vi "Config Sequence.vi"(8 "error in (no error)":errorcluster, 10 "new element/subarray":refnum<class "STEP.lvclass">, 11 "All Sequence STEPs in":refnum<class "STEP.lvclass">[](array[class])) -> (0 "error out":errorcluster, 3 "All Sequence STEPs":refnum<class "STEP.lvclass">[](array[class]))   [LabVIEW 2014, in "SeqLoop.lvlib"]
doc: "Configura las Mediciones."
uses:
  SeqLoop.lvlib
  Classes/STEP/STEP.lvclass
  <vilib>/regexp/Match Regular Expression.xnode
panel:
  in  "Ver Seq":bool
  in  "Stop Seq":bool
  in  "Delete Seq":bool
  in  "Add Seq":bool
  in  "Secuencias":i32(listbox)=-1 caption="Secuencia"
  in  "Edit Seq":bool
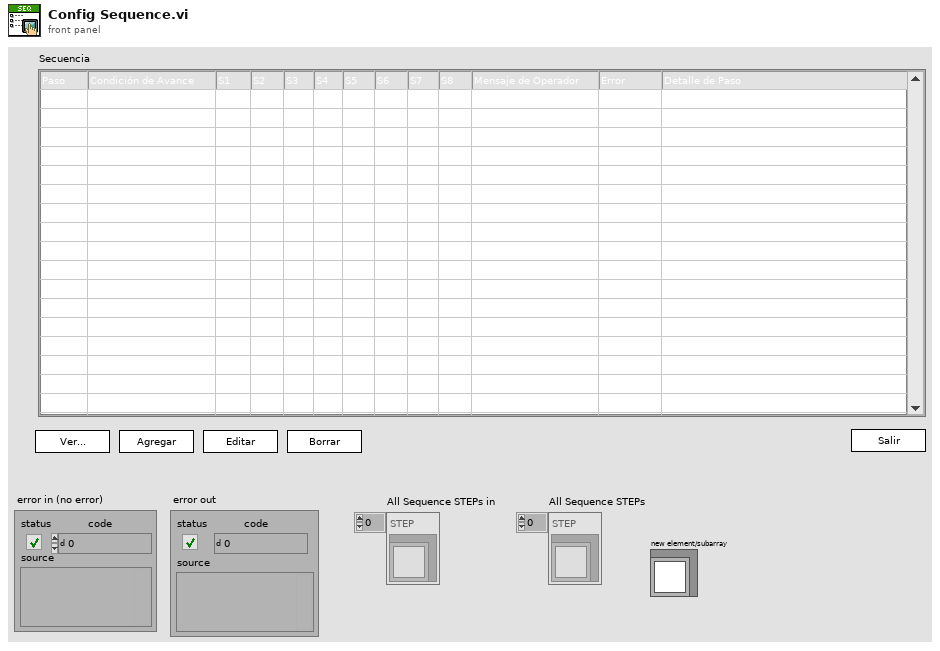
[diagram p1: front panel]
types:
  T1 = enum8{"Enabled", "Disabled", "Disabled and Grayed Out"}
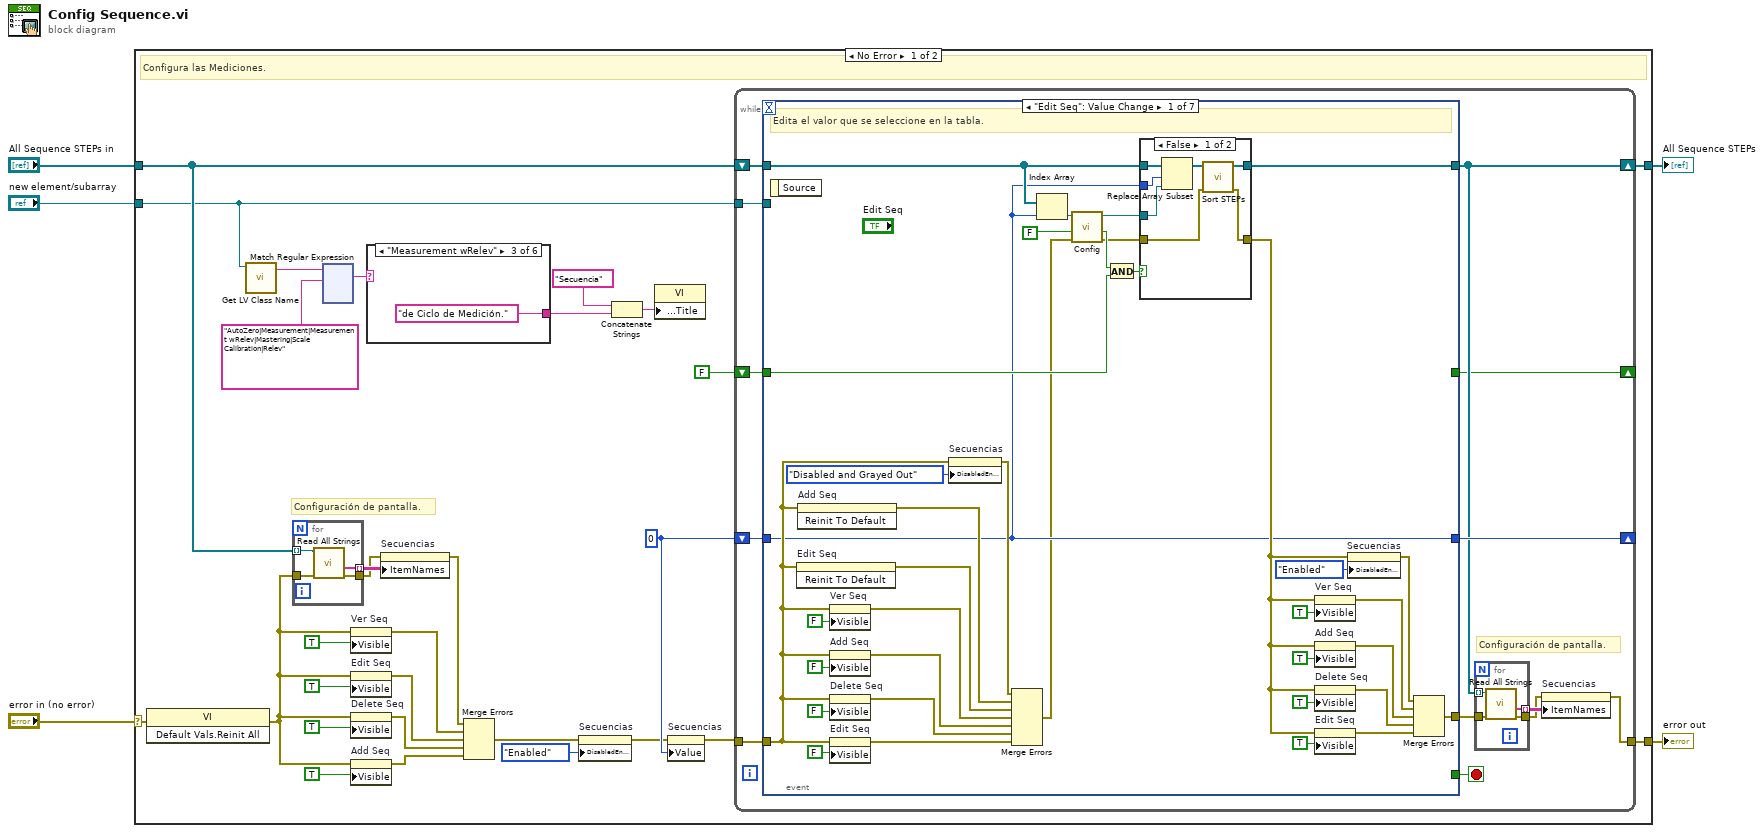
[diagram p0: block diagram]
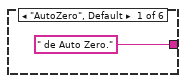
[diagram p2: hidden frame]
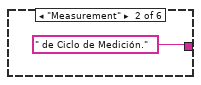
[diagram p3: hidden frame]
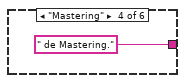
[diagram p4: hidden frame]
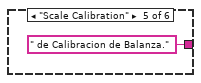
[diagram p5: hidden frame]
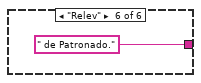
[diagram p6: hidden frame]
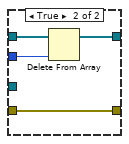
[diagram p7: hidden frame]
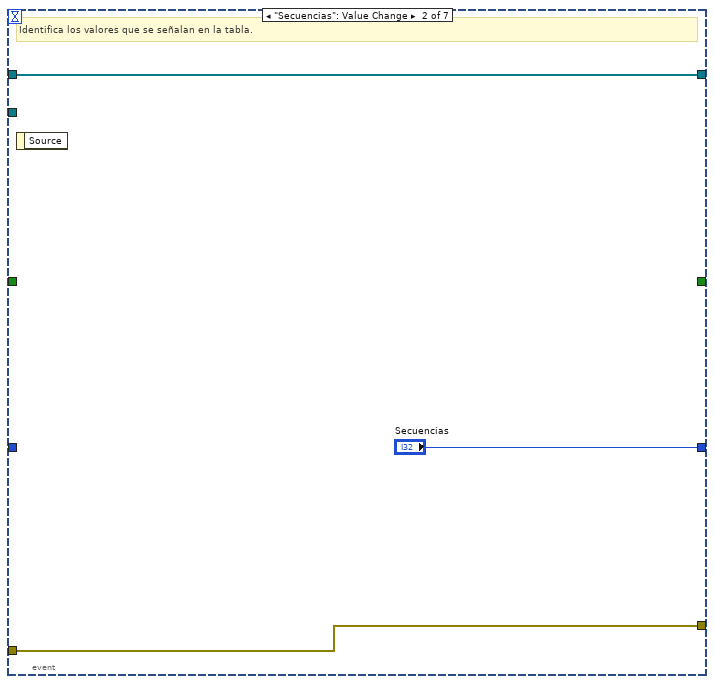
[diagram p8: hidden frame]
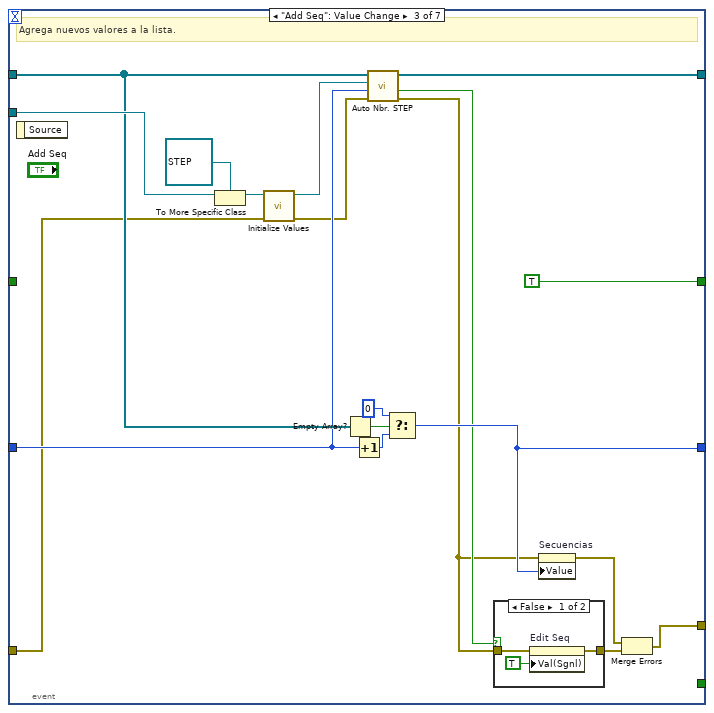
[diagram p9: hidden frame]
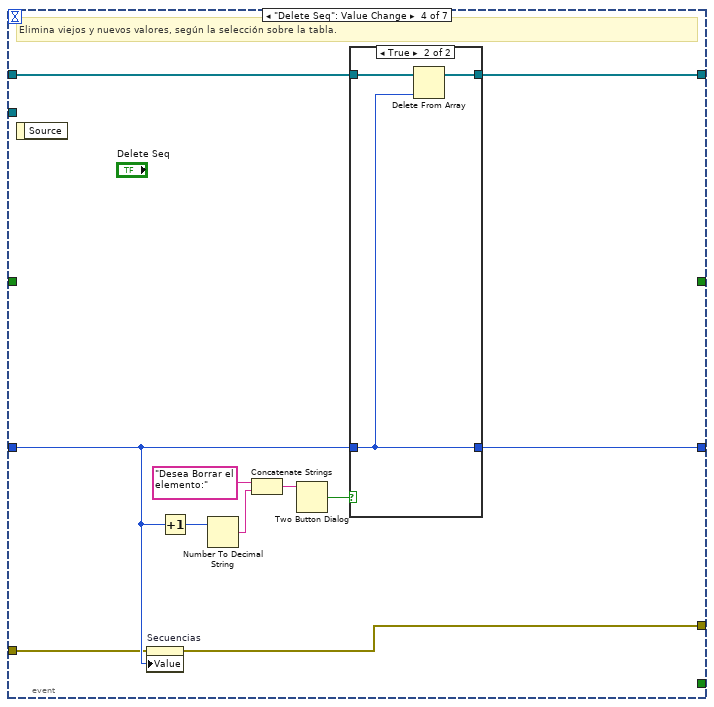
[diagram p11: hidden frame]
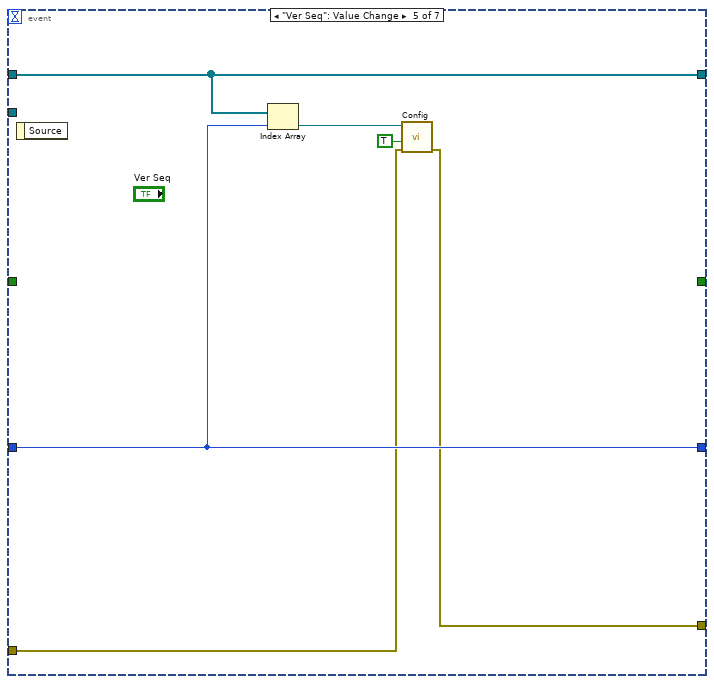
[diagram p13: hidden frame]
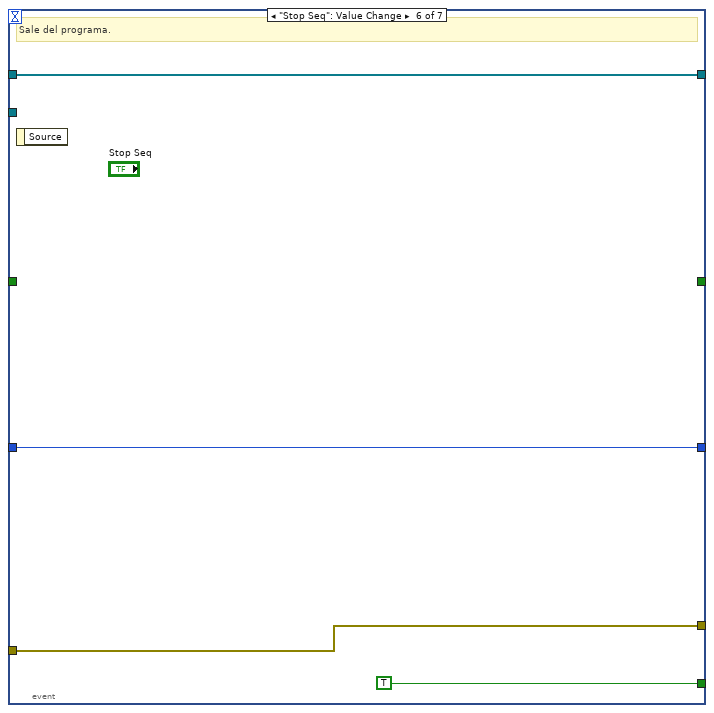
[diagram p14: hidden frame]
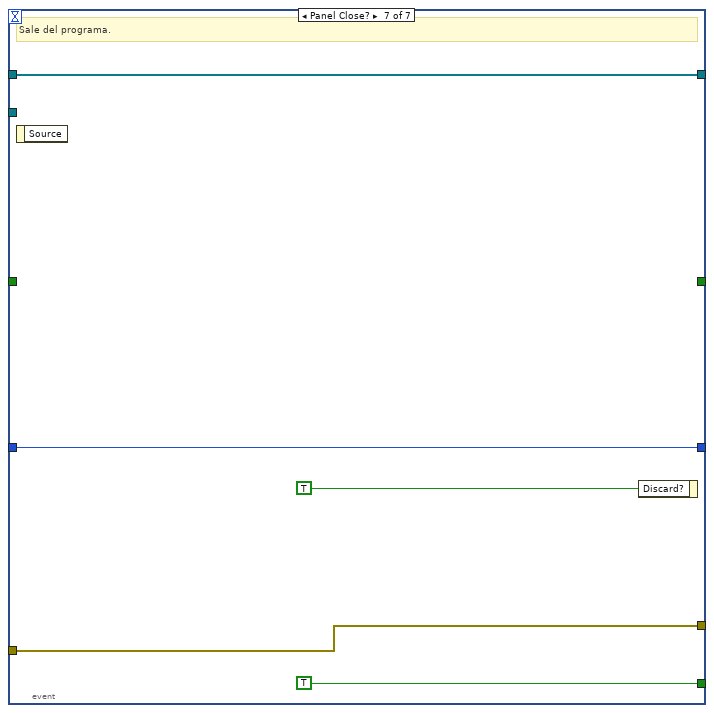
[diagram p15: hidden frame]
diagram:
  n1 = case shown="No Error" "error in (no error)" {
    selector: "error in (no error)" -> [w21 w280]
    tunnel: [w34 w280] -> w5
    tunnel: [w27 w281] -> w3
    tunnel: "All Sequence STEPs in" -> [w26 w281]
    tunnel: "new element/subarray" -> [w12 _]
    frame No Error {
      w23 = 0 ("disabled index (col)")
      # "Configuración de pantalla."
      # "Configura las Mediciones."
      n2 = invoke class="VI" method="Default Vals.Reinit All"(error in=w21) -> (error out=w16:errorcluster)  [unwired: 2 in, 2 out]
      n3 = call <vilib>:"Get LV Class Name.vi"("object"=w12) -> ("class name"=w11:string)  [unwired: 9 in, 1 out]
      n4 = for {
        tunnel: w26 -> [w158] mode=indexing
        tunnel: w16 -> [w156]
        tunnel: [w157] -> w25 mode=indexing
        tunnel: [w155] -> w24
        n5 = call "Read All Strings.vi"("error in (no error)"=w156, "STEP in"=w158) -> ("error out"=w155:errorcluster, "All Strings"=w157:string[])  [unwired: 7 in, 1 out]
      }
      n6 = xnode "Match Regular Expression"("input string"=w11, "regular expression"="AutoZero|Measurement|Measurement wRelev|Mastering|Scale Calibration|Relev") -> ("whole match"=w9:string)  [unwired: 4 in, 4 out]
      n7 = property on="Ver Seq" class="Bool"(error in=w16, "Visible"=TRUE) -> (error out=w15:errorcluster)  [unwired: 1 in, 1 out]
      n8 = property on="Edit Seq" class="Bool (strict)"(error in=w16, "Visible"=TRUE) -> (error out=w32:errorcluster)  [unwired: 1 in, 1 out]
      n9 = property on="Delete Seq" class="Bool"(error in=w16, "Visible"=TRUE) -> (error out=w30:errorcluster)  [unwired: 1 in, 1 out]
      n10 = property on="Add Seq" class="Bool (strict)"(error in=w16, "Visible"=TRUE) -> (error out=w28:errorcluster)  [unwired: 1 in, 1 out]
      n11 = case shown="\"Measurement wRelev\"" w9 {
        tunnel: [" de Auto Zero." ("Program Type") " de Ciclo de Medición." ("Program Type") "de Ciclo de Medición." ("Program Type") " de Mastering." ("Program Type") " de Calibracion de Balanza." ("Program Type") " de Patronado." ("Program Type")] -> w6
        frame "AutoZero", Default {
        }
        frame "Measurement" {
        }
        frame "Measurement wRelev" {
        }
        frame "Mastering" {
        }
        frame "Scale Calibration" {
        }
        frame "Relev" {
        }
      }
      n12 = property on="Secuencias" class="MCListbox (strict)"(error in=w24, "ItemNames"=w25) -> (error out=w14:errorcluster)  [unwired: 1 in, 1 out]
      n13 = Merge Errors(w14, w15, w32, w30, w28) -> (w20:errorcluster)
      n14 = property on="Secuencias" class="MCListbox (strict)"(error in=w20, "DisabledEnum"=T1."Enabled" ("Disabled")) -> (error out=w19:errorcluster)  [unwired: 1 in, 1 out]
      n15 = Concatenate Strings("Secuencia" ("Program Type"), w6) -> (w8:string)
      n16 = property class="VI"("Front Panel.Title"=w8) -> ()  [unwired: 2 in, 2 out]
      n17 = property on="Secuencias" class="MCListbox (strict)"(error in=w19, "Value"=w23) -> (error out=w18:errorcluster)  [unwired: 1 in, 1 out]
      n18 = while {
        shift-right: [w166] -> w27
        shift-left: w26 -> [w167]
        shift-right: [w168] -> _
        shift-left: w23 -> [w169]
        tunnel: w18 -> [w171]
        tunnel: [w162] -> w34
        tunnel: w12 -> [w161]
        shift-right: [w160] -> _
        shift-left: FALSE -> [w159]
        stop <- w170 stop-if-true
        # "Configuración de pantalla."
        n19 = event shown="[0] \"Edit Seq\": Value Change" {
          selector: _ -> [_ _ _ _ _ _ _]
          dyn-events: _ -> [_ _ _ _ _ _ _]
          timeout: _ -> [_ _ _ _ _ _ _]
          tunnel: w167 -> [w182 w225 w235 w257 w270 w273 w279]
          tunnel: [w204 w225 w237 w256 w270 w273 w279] -> w166
          tunnel: [w181 "Secuencias" w230 w258 w269 w272 w278] -> w168
          tunnel: w169 -> [w181 _ w232 w251 w269 w272 w278]
          tunnel: w171 -> [w205 w223 w227 w250 w268 w274 w276]
          tunnel: [w187 w223 w242 w249 w267 w274 w276] -> w164
          tunnel: [_ _ _ _ _ TRUE ("Stop Med") TRUE ("Stop Med")] -> w170
          tunnel: w161 -> [_ _ w240 _ _ _ _]
          tunnel: [_ _ TRUE _ _ _ _] -> w160
          tunnel: w159 -> [w185 _ _ _ _ _ _]
          event "Edit Seq": Value Change {
            # "Edita el valor que se seleccione en la tabla."
            n20 = event-data() -> ()  [unwired: 1 in, 1 out]
            n21 = invoke on="Edit Seq" class="Bool (strict)" method="Reinit To Default"(error in=w205) -> (error out=w201:errorcluster)  [unwired: 2 in, 2 out]
            n22 = invoke on="Add Seq" class="Bool (strict)" method="Reinit To Default"(error in=w205) -> (error out=w200:errorcluster)  [unwired: 2 in, 2 out]
            n23 = property on="Ver Seq" class="Bool"(error in=w205, "Visible"=FALSE) -> (error out=w203:errorcluster)  [unwired: 1 in, 1 out]
            n24 = property on="Add Seq" class="Bool (strict)"(error in=w205, "Visible"=FALSE) -> (error out=w208:errorcluster)  [unwired: 1 in, 1 out]
            n25 = property on="Delete Seq" class="Bool"(error in=w205, "Visible"=FALSE) -> (error out=w202:errorcluster)  [unwired: 1 in, 1 out]
            n26 = property on="Edit Seq" class="Bool (strict)"(error in=w205, "Visible"=FALSE) -> (error out=w198:errorcluster)  [unwired: 1 in, 1 out]
            n27 = property on="Secuencias" class="MCListbox (strict)"(error in=w205, "DisabledEnum"=T1."Disabled and Grayed Out" ("Disabled")) -> (error out=w199:errorcluster)  [unwired: 1 in, 1 out]
            n28 = Merge Errors(w199, w200, w201, w203, w208, w202, w198) -> (w180:errorcluster)
            n29 = Index Array(array=w182, index=w181) -> (element=w179:refnum<class "STEP.lvclass">)
            n30 = call "Config.vi"("error in (no error)"=w180, "Read only?"=FALSE ("View?"), "STEP in"=w179) -> ("error out"=w176:errorcluster, "Discard?"=w177:bool, "STEP out"=w178:refnum<class "STEP.lvclass">)  [unwired: 6 in]
            n31 = And(x=w177, y=w185) -> (x .and. y?=w184:bool)
            n32 = case shown="False" w184 {
              tunnel: w182 -> [w218 w221]
              tunnel: w181 -> [w217 w219]
              tunnel: w178 -> [w216 _]
              tunnel: [w214 w220] -> w204
              tunnel: w176 -> [w213 w222]
              tunnel: [w212 w222] -> w188
              frame False {
                n33 = Replace Array Subset(array=w218, new element=w216, index=w217) -> (w215:refnum<class "STEP.lvclass">[])
                n34 = call "Sort STEPs.vi"("error in (no error)"=w213, "All Sequence STEPs in"=w215) -> ("error out"=w212:errorcluster, "All Sequence STEPs"=w214:refnum<class "STEP.lvclass">[])  [unwired: 8 in]
              }
              frame True {
                n35 = Delete From Array(array=w221, index=w219) -> (array with subset deleted=w220:refnum<class "STEP.lvclass">[])  [unwired: 1 in, 1 out]
              }
            }
            n36 = property on="Ver Seq" class="Bool"(error in=w188, "Visible"=TRUE) -> (error out=w195:errorcluster)  [unwired: 1 in, 1 out]
            n37 = property on="Add Seq" class="Bool (strict)"(error in=w188, "Visible"=TRUE) -> (error out=w192:errorcluster)  [unwired: 1 in, 1 out]
            n38 = property on="Delete Seq" class="Bool"(error in=w188, "Visible"=TRUE) -> (error out=w196:errorcluster)  [unwired: 1 in, 1 out]
            n39 = property on="Edit Seq" class="Bool (strict)"(error in=w188, "Visible"=TRUE) -> (error out=w197:errorcluster)  [unwired: 1 in, 1 out]
            n40 = property on="Secuencias" class="MCListbox (strict)"(error in=w188, "DisabledEnum"=T1."Enabled" ("Disabled")) -> (error out=w186:errorcluster)  [unwired: 1 in, 1 out]
            n41 = Merge Errors(w186, w195, w192, w196, w197) -> (w187:errorcluster)
          }
          event "Secuencias": Value Change {
            # "Identifica los valores que se señalan en la tabla."
            n42 = event-data() -> ()  [unwired: 1 in, 1 out]
          }
          event "Add Seq": Value Change {
            # "Agrega nuevos valores a la lista."
            n43 = event-data() -> ()  [unwired: 1 in, 1 out]
            n44 = To More Specific Class(target class=refnum<class "STEP.lvclass"> refnum, reference=w240) -> (specific class reference=w241:refnum<class "STEP.lvclass">)  [unwired: 1 in, 1 out]
            n45 = call-dynamic "Initialize Values.vi"("error in (no error)"=w227, "STEP in"=w241) -> ("error out"=w228:errorcluster, "STEP out"=w236:refnum<class "STEP.lvclass">)  [unwired: 8 in]
            n46 = Empty Array?(array=w235) -> (empty?=w234:bool)
            n47 = Increment(x=w232) -> (x+1=w231:i32)
            n48 = call "Auto Nbr. STEP.vi"("error in (no error)"=w228, "index (col)"=w232, "STEP in"=w236, "All Sequence STEPs in"=w235) -> ("error out"=w226:errorcluster, "Discarded?"=w229:bool, "All Sequence STEPs out"=w237:refnum<class "STEP.lvclass">[])  [unwired: 5 in]
            n49 = Select(t=0 ("disabled index (col)"), s=w234, f=w231) -> (s? t:f=w230:i32)
            n50 = case shown="False" w229 {
              tunnel: [w247 w248] -> w244
              tunnel: w226 -> [w246 w248]
              frame False {
                n51 = property on="Edit Seq" class="Bool (strict)"(error in=w246, "Val(Sgnl)"=TRUE ("Value (Signaling)")) -> (error out=w247:errorcluster)  [unwired: 1 in, 1 out]
              }
              frame True {
              }
            }
            n52 = property on="Secuencias" class="MCListbox (strict)"(error in=w226, "Value"=w230) -> (error out=w243:errorcluster)  [unwired: 1 in, 1 out]
            n53 = Merge Errors(w243, w244) -> (w242:errorcluster)
          }
          event "Delete Seq": Value Change {
            # "Elimina viejos y nuevos valores, según la selección sobre la tabla."
            n54 = event-data() -> ()  [unwired: 1 in, 1 out]
            n55 = property on="Secuencias" class="MCListbox (strict)"(error in=w250, "Value"=w251) -> (error out=w249:errorcluster)  [unwired: 1 in, 1 out]
            n56 = Increment(x=w251) -> (x+1=w252:i32)
            n57 = Number To Decimal String(number=w252) -> (decimal integer string=w254:string)  [unwired: 1 in]
            n58 = Concatenate Strings("Desea Borrar el elemento:" ("message"), w254) -> (w253:string)
            n59 = Two Button Dialog(message=w253) -> (T button?=w259:bool)  [unwired: 2 in]
            n60 = case shown="True" w259 {
              tunnel: w257 -> [w260 w264]
              tunnel: [w261 w262] -> w258
              tunnel: w251 -> [w261 w262]
              tunnel: [w260 w263] -> w256
              frame False {
              }
              frame True {
                n61 = Delete From Array(array=w264, index=w262) -> (array with subset deleted=w263:refnum<class "STEP.lvclass">[])  [unwired: 1 in, 1 out]
              }
            }
          }
          event "Ver Seq": Value Change {
            n62 = event-data() -> ()  [unwired: 1 in, 1 out]
            n63 = Index Array(array=w270, index=w269) -> (element=w265:refnum<class "STEP.lvclass">)
            n64 = call "Config.vi"("error in (no error)"=w268, "Read only?"=TRUE ("View?"), "STEP in"=w265) -> ("error out"=w267:errorcluster)  [unwired: 6 in, 2 out]
          }
          event "Stop Seq": Value Change {
            # "Sale del programa."
            n65 = event-data() -> ()  [unwired: 1 in, 1 out]
          }
          event Panel Close? {
            # "Sale del programa."
            n66 = event-data() -> ()  [unwired: 1 in, 1 out]
            n67 = event-data("Discard?"=TRUE) -> ()  [unwired: 1 in, 1 out]
          }
        }
        n68 = for {
          tunnel: w166 -> [w175] mode=indexing
          tunnel: w164 -> [w173]
          tunnel: [w174] -> w165 mode=indexing
          tunnel: [w172] -> w163
          n69 = call "Read All Strings.vi"("error in (no error)"=w173, "STEP in"=w175) -> ("error out"=w172:errorcluster, "All Strings"=w174:string[])  [unwired: 7 in, 1 out]
        }
        n70 = property on="Secuencias" class="MCListbox (strict)"(error in=w163, "ItemNames"=w165) -> (error out=w162:errorcluster)  [unwired: 1 in, 1 out]
      }
    }
    frame Error {
    }
  }
  "error out" <- w5
  "All Sequence STEPs" <- w3
